vi "free Field.vi"(11 "field":T1) -> (3 "field out":T1)   [LabVIEW 2012, in "Lightpipes.lvlib"]
doc: "__declspec(dllexport) void free_field(FIELD* field);"
uses:
  LightPipes.lvlib
  Lightpipes.dll
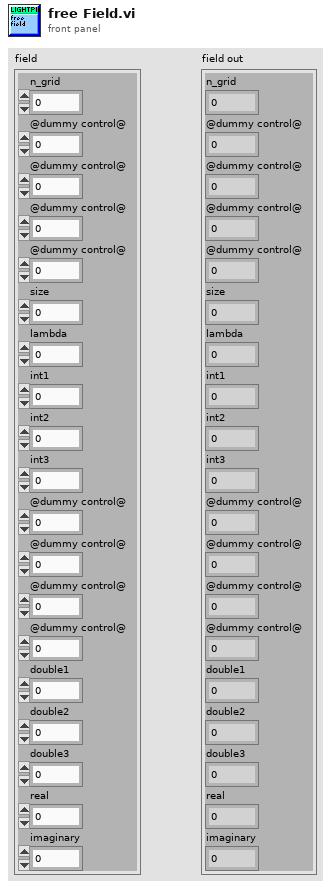
[diagram p1: front panel]
types:
  T1 = cluster{"n_grid":i32, "@dummy control@":i8, "@dummy control@":i8, "@dummy control@":i8, "@dummy control@":i8, "size":dbl, "lambda":dbl, "int1":i32, "int2":i32, "int3":i32, "@dummy control@":i8, "@dummy control@":i8, "@dummy control@":i8, "@dummy control@":i8, "double1":dbl, "double2":dbl, "double3":dbl, "real":u32, "imaginary":u32}
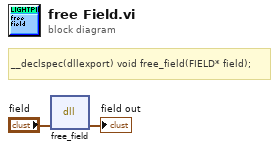
[diagram p0: block diagram]
diagram:
  # "__declspec(dllexport) void free_field(FIELD* field);"
  n1 = dll-call lib="C:/Users/Tri/Documents/Gerchberg/Lightpipes.*" fn="free_field"("field"="field") -> ("field"=→"field out":T1)  [unwired: 4 in, 2 out]
